vi "BuildParamsMsg.vi"(0 "Parameters":cluster{"Joint":string, "value":dbl}[](array[cluster])) -> (2 "Commands":string[](array[string]))   [LabVIEW 2012]
doc: "Converts joint parameters to commands"
uses:
  <userlib>/ROSforLV/ROS/MessageBuilding/std_msgs/subs/float64Array.vi
  <userlib>/ROSforLV/ROS/MessageBuilding/std_msgs/subs/stringArray.vi
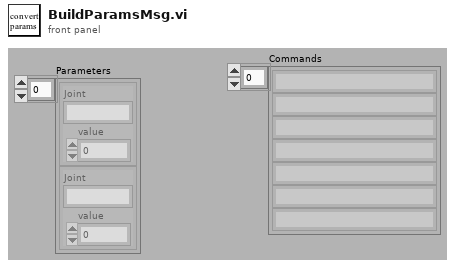
[diagram p1: front panel]
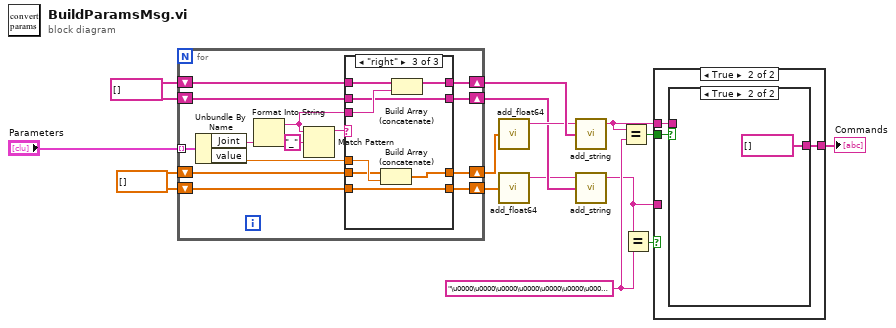
[diagram p0: block diagram]
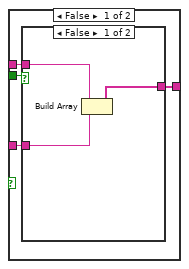
[diagram p2: hidden frame]
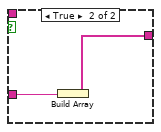
[diagram p3: hidden frame]
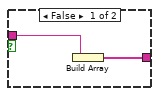
[diagram p4: hidden frame]
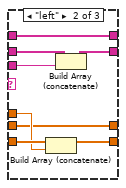
[diagram p6: hidden frame]
diagram:
  w5 = "\u0000\u0000\u0000\u0000\u0000\u0000\u0000\u0000" ("left msg")
  w11 = dbl[] []
  w12 = string[] []
  n1 = for {
    shift-right: [w26] -> w9
    shift-left: w12 -> [w29]
    shift-right: [w27] -> w10
    shift-left: w11 -> [w28]
    tunnel: "Parameters" -> [w25] mode=indexing
    shift-right: [w18] -> w15
    shift-left: w12 -> [w19]
    shift-right: [w16] -> w14
    shift-left: w11 -> [w17]
    n2 = Unbundle By Name(w25) -> ("Joint"=w22:string, "value"=w24:dbl)
    n3 = Format Into String(w22) -> (resulting string=w23:string)  [unwired: 3 in, 1 out]
    n4 = Match Pattern(string=w23, regular expression="_") -> (before substring=w20:string)  [unwired: 1 in, 3 out]
    n5 = case shown="\"right\"" w20 {
      tunnel: w29 -> [w33 w41 w45]
      tunnel: w28 -> [w32 w39 w42]
      tunnel: [w32 w38 w42] -> w27
      tunnel: [w33 w40 w45] -> w26
      tunnel: w24 -> [_ w37 w49]
      tunnel: w23 -> [_ w36 w48]
      tunnel: w19 -> [w31 w35 w47]
      tunnel: [w31 w35 w46] -> w18
      tunnel: w17 -> [w30 w34 w44]
      tunnel: [w30 w34 w43] -> w16
      frame Default {
      }
      frame "left" {
        n6 = Build Array (concatenate)(w39, w37) -> (w38:dbl[])
        n7 = Build Array (concatenate)(w41, w36) -> (w40:string[])
      }
      frame "right" {
        n8 = Build Array (concatenate)(w44, w49) -> (w43:dbl[])
        n9 = Build Array (concatenate)(w47, w48) -> (w46:string[])
      }
    }
  }
  n10 = call-poly <userlib>:"add_float64.vi"("Array"=w14) -> ("msg out"=w13:string)  [unwired: 4 in]
  n11 = call-poly <userlib>:"add_float64.vi"("Array"=w10) -> ("msg out"=w8:string)  [unwired: 4 in]
  n12 = call-poly <userlib>:"add_string.vi"("Array"=w15, "msg in"=w13) -> ("msg out"=w3:string)  [unwired: 3 in]
  n13 = call-poly <userlib>:"add_string.vi"("Array"=w9, "msg in"=w8) -> ("msg out"=w2:string)  [unwired: 3 in]
  n14 = Equal?(x=w3, y=w5) -> (x = y?=w4:bool)
  n15 = Equal?(x=w2, y=w5) -> (x = y?=w6:bool)
  n16 = case shown="True" w6 {
    tunnel: w4 -> [w53 w61]
    tunnel: w3 -> [w50 w60]
    tunnel: [w51 w59] -> w1
    tunnel: w2 -> [w52 _]
    frame False {
      n17 = case shown="False" w53 {
        tunnel: w52 -> [w55 w58]
        tunnel: [w54 w57] -> w51
        tunnel: w50 -> [w56 _]
        frame False {
          n18 = Build Array(w56, w55) -> (w54:string[])
        }
        frame True {
          n19 = Build Array(w58) -> (w57:string[])
        }
      }
    }
    frame True {
      n20 = case shown="True" w61 {
        tunnel: w60 -> [w63 _]
        tunnel: [w62 string[] []] -> w59
        frame False {
          n21 = Build Array(w63) -> (w62:string[])
        }
        frame True {
        }
      }
    }
  }
  "Commands" <- w1
